vi "Set Bar Color.vi"(8 "error in (no error)":errorcluster, 10 "Bar Color":u32(colorbox)) -> (0 "error out":errorcluster)   [LabVIEW 2013, in "Progress Bar.lvlib"]
uses:
  Progress Bar.lvlib
  Queue/Queue Action.ctl
  Queue/Property Message.ctl
  Queue/Property Action.ctl
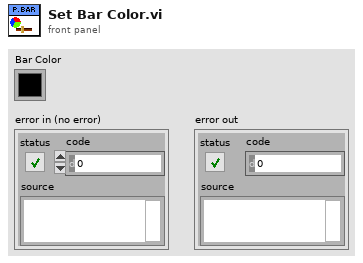
[diagram p1: front panel]
types:
  T1 = typedef "Progress Bar.lvlib/Property Message.ctl" = cluster{"Property":T2, "Value":variant}
  T2 = typedef "Progress Bar.lvlib/Property Action.ctl" = enum16{"BG Color", "Title Text Color", "Title Text", "Action Text Color", "Action Text", "Bar Color", "Set Slider Value", "Add to Slider Value", "Exit"}
  T3 = typedef "Progress Bar.lvlib/Queue Action.ctl" = enum16{"Obtain Queue", "Release Queue", "Get Queue"}
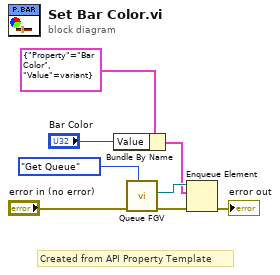
[diagram p0: block diagram]
diagram:
  # "Created from API Property Template"
  n1 = Bundle By Name(cluster=T1 {"Property"=enum."Bar Color", "Value"=variant} ("element"), "Value"="Bar Color") -> (w4:T1)
  n2 = call "Queue FGV.vi"("Enum"=Queue_Action."Get Queue", "error in (no error)"="error in (no error)") -> ("error out"=w1:errorcluster, "queue out"=w7:refnum<queue>)  [unwired: 8 in]
  n3 = Enqueue Element(queue=w7, element=w4, error in (no error)=w1) -> (error out=→"error out":errorcluster)  [unwired: 1 in, 2 out]
